vi "OnOffArray.vi"(11 "Size":i32) -> (3 "OnOffAr":enum16{"On", "Off"}[](array[ring]))   [LabVIEW 2014]
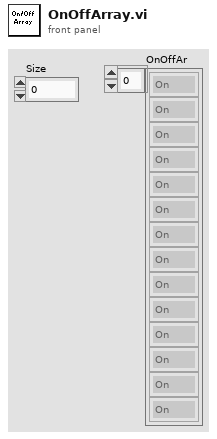
[diagram p1: front panel]
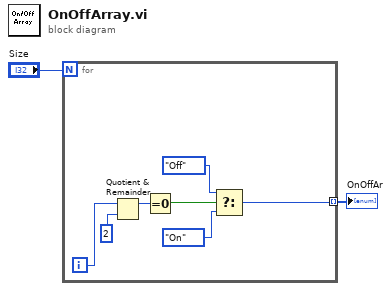
[diagram p0: block diagram]
diagram:
  n1 = for {
    N: "Size" -> [_]
    tunnel: [w3] -> w1 mode=indexing
    i -> [w9]
    n2 = Quotient & Remainder(x=w9, y=2) -> (x-y*floor(x/y)=w7:i32)  [unwired: 1 out]
    n3 = Equal To 0?(x=w7) -> (x = 0?=w6:bool)
    n4 = Select(t=enum16{"On", "Off"}."Off", s=w6, f=enum16{"On", "Off"}."On") -> (s? t:f=w3:enum16{"On", "Off"})
  }
  "OnOffAr" <- w1
